vi "Untitled 1.vi"() -> ()   [LabVIEW 2024]
panel:
  in  "G":dbl
  in  "k_i":dbl
  in  "T":dbl
  in  "I_sc":dbl
  out "I_ph":dbl
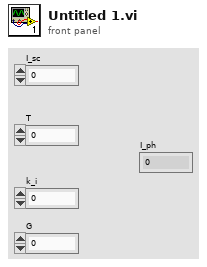
[diagram p1: front panel]
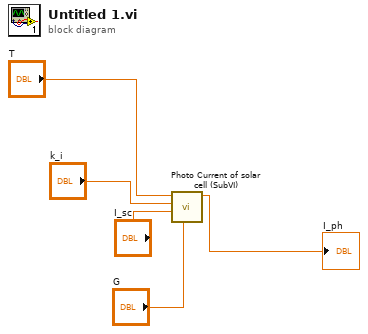
[diagram p0: block diagram]
diagram:
  n1 = call "Photo Current of solar cell (SubVI).vi"("G"="G", "I_sc"="I_sc", "k_i"="k_i", "T"="T") -> ("I_ph"=→"I_ph":dbl)  [unwired: 7 in]
